vi "Inverse Time Curves (IEEE, Dependent Reset).vi"(6 "operate time compensation":cluster{"G/Gs":dbl, "compensation [s]":dbl}[](array[cluster]), 7 "GD (25)":u16=25, 8 "error in (no error)":errorcluster, 10 "time multiplier setting (1)":dbl=1.0, 11 "curve type":u16(ring) items=["IEEE moderately inverse", "IEEE very inverse", "IEEE extremely inverse"]) -> (0 "error out":errorcluster, 2 "memory size":u16, 3 "memory initial values":fxp<+,51,51>[](array[numeric]), 4 "curve data":cluster{"G/Gs":dbl[], "times [s]":dbl[]})   [LabVIEW 2014, in "NI_EP_Protection.lvlib"]
doc: "Generates memory initial values and memory size, which contain the information of the inverse time curves, for the FPGA Inverse Time Delay VI to use. You can compensate for the processing delay of the input energizing quantity under a specific G/Gs to achieve higher operate time accuracy."
uses:
  <vilib>/addons/Electrical Power/Protection/NI_EP_Protection.lvlib
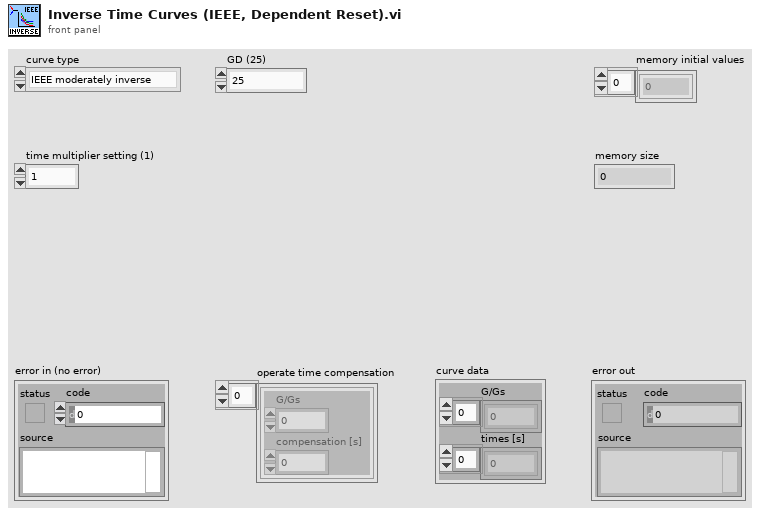
[diagram p1: front panel]
types:
  T1 = typedef "NI_EP_Protection.lvlib/ep_Curve Parameters.ctl" = cluster{"operate time parameters":T2, "reset time parameters":T3}
  T2 = typedef "NI_EP_Protection.lvlib/ep_Operate Time.ctl" = cluster{"A [s]":dbl, "B [s]":dbl, "alpha":dbl, "K2 [s]":dbl, "K1 [s]":dbl, "K3 [s]":dbl}
  T3 = typedef "NI_EP_Protection.lvlib/ep_Reset Time.ctl" = cluster{"tr [s]":dbl, "alpha":dbl}
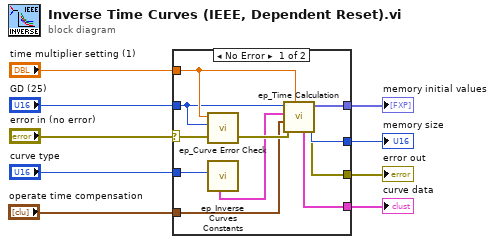
[diagram p0: block diagram]
diagram:
  n1 = case shown="No Error" "error in (no error)" {
    selector: "error in (no error)" -> [w18 w21]
    tunnel: [w13 w21] -> w8
    tunnel: "curve type" -> [w15 _]
    tunnel: "GD (25)" -> [w19 _]
    tunnel: "time multiplier setting (1)" -> [w20 _]
    tunnel: [w16 _] -> w4
    tunnel: [w14 _] -> w3
    tunnel: [w12 _] -> w2
    tunnel: "operate time compensation" -> [w10 _]
    frame No Error {
      n2 = call <vilib>:"ep_Curve Error Check.vi"("error in (no error)"=w18, "GD"=w19, "time dial"=w20) -> ("error out"=w17:errorcluster)  [unwired: 8 in]
      n3 = call <vilib>:"ep_Inverse Curves Constants.vi"("IEEE curve type"=w15) -> ("IEEE parameters"=w11:T1)  [unwired: 5 in, 5 out]
      n4 = call <vilib>:"ep_Time Calculation.vi"("time dial"=w20, "error in (no error)"=w17, "operate time compensation"=w10, "curve parameters"=w11, "GD"=w19) -> ("error out"=w13:errorcluster, "memory size"=w16:u16, "memory initial values"=w14:fxp<+,51,51>[], "curve data"=w12:cluster{"G/Gs":dbl[], "times":dbl[]})  [unwired: 3 in]
    }
    frame Error {
    }
  }
  "memory initial values" <- w3
  "error out" <- w8
  "memory size" <- w4
  "curve data" <- w2
